vi "GetValidMoves.vi"(1 "Board":i32[][](array[numeric])) -> (0 "Vaild moves":bool[](array[boolean]))   [LabVIEW 2025]
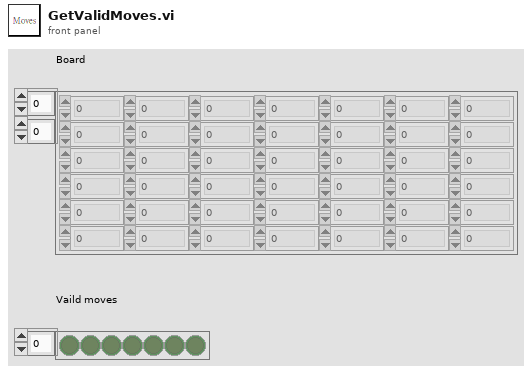
[diagram p1: front panel]
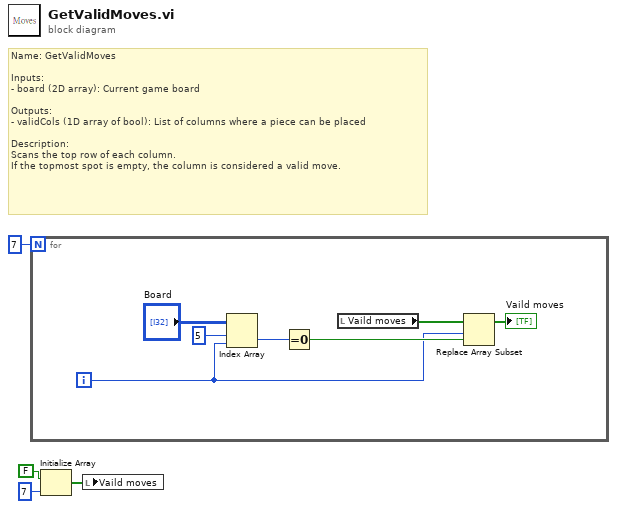
[diagram p0: block diagram]
diagram:
  # "Name: GetValidMoves\n\nInputs:\n- board (2D array): Current game board\n\nOutputs:\n- validCols (1D array of bool): List of columns where a piece can be placed\n\nDescription:\nScans the top row of each column.\nIf the topmost spot is empty, the column is considered a valid move."
  n1 = for {
    N: 7 -> [_]
    i -> [w5]
    n2 = Index Array(array="Board", index (row)=5, index (col)=w5) -> (element=w7:i32)
    n3 = Equal To 0?(x=w7) -> (x = 0?=w8:bool)
    n4 = local read "Vaild moves"() -> (w10:bool[])
    n5 = Replace Array Subset(array=w10, new element=w8, index=w5) -> (→"Vaild moves":bool[])
  }
  n6 = Initialize Array(FALSE, 7 ("dimension size")) -> (w3:bool[])
  n7 = local write "Vaild moves"(w3) -> ()
